vi "st_Is NaN or Inf.vi"(4 "x":dbl) -> (1 "isNaN(x) || isInf(x)":bool)   [LabVIEW 2017, in "NI_Gmath.lvlib"]
uses:
  <vilib>/gmath/NI_Gmath.lvlib
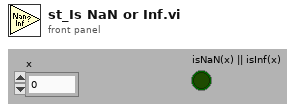
[diagram p1: front panel]
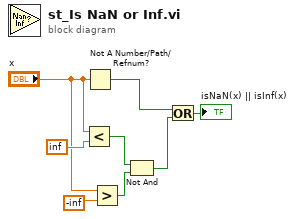
[diagram p0: block diagram]
diagram:
  n1 = Less?(x="x", y=inf) -> (x < y?=w5:bool)
  n2 = Not A Number/Path/Refnum?(number/path/refnum="x") -> (NaN/Path/Refnum?=w2:bool)
  n3 = Greater?(x="x", y=-inf) -> (0:w4:bool)
  n4 = Not And(1:w4, 2:w5) -> (0:w3:bool)
  n5 = Or(x=w2, y=w3) -> (x .or. y?=→"isNaN(x) || isInf(x)":bool)
